vi "Create Handle Activate Menu On Tree Item Msg.vi"(7 "Return Priority (Normal)":T1=enum."Normal", 11 "Return Enqueuer":refnum<class "Message Enqueuer.lvclass">) -> (3 "Handle Activate Menu On Tree Item Msg out":refnum<class "Handle Activate Menu On Tree Item Msg.lvclass">)   [LabVIEW 2020, in "File Explorer.lvlib" / "Handle Activate Menu On Tree Item Msg.lvclass"]
uses:
  <vilib>/gpm_packages/@cs/file-explorer-extension/Source/File Explorer/File Explorer Messages/Handle Activate Menu On Tree Item Msg/Handle Activate Menu On Tree Item Msg.lvclass
  C:/Program Files/National Instruments/LabVIEW 2020/vi.lib/gpm_packages/@cs/actor-framework-messages/Source/RoundTripMessage/RoundTripMessage.lvclass
  <vilib>/ActorFramework/Message Enqueuer/Message Enqueuer.lvclass
  <vilib>/ActorFramework/Message Enqueuer/Message Priority.ctl
  <vilib>/gpm_packages/@cs/actor-framework-messages/Source/RoundTripMessage/RoundTripMessage.lvclass/RoundTripMessage.ctl
  <vilib>/gpm_packages/@cs/actor-framework-messages/Source/RoundTripMessage/RoundTripMessage.lvclass
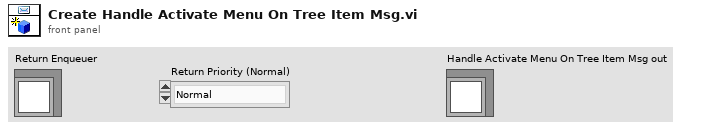
[diagram p1: front panel]
types:
  T1 = typedef "Actor Framework.lvlib/Message Enqueuer.lvclass/Message Priority.ctl" = enum16{"Low", "Normal", "High"}
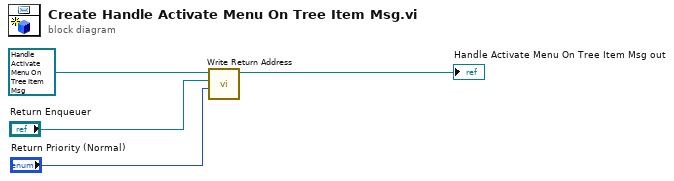
[diagram p0: block diagram]
diagram:
  n1 = call <vilib>:"Write Return Address.vi"("Return Priority (Normal)"="Return Priority (Normal)", "Return Enqueuer"="Return Enqueuer", "RoundTripMessage In"=refnum<class "Handle Activate Menu On Tree Item Msg.lvclass"> refnum ("Handle Activate Menu On Tree Item Msg in")) -> ("RoundTripMessage Out"=→"Handle Activate Menu On Tree Item Msg out":refnum<class "Handle Activate Menu On Tree Item Msg.lvclass">)  [unwired: 8 in]
